vi "AFM_Driver_Manager.DestroyEvents.vi"(8 "error in (no error)":errorcluster, 11 "AFM_Driver_Manager in":refnum<class "AFM_Driver_Manager.lvclass">) -> (0 "error out":errorcluster, 3 "AFM_Driver_Manager out":refnum<class "AFM_Driver_Manager.lvclass">)   [LabVIEW 2019, in "AFM_Driver_Manager.lvclass"]
uses:
  AFM_Driver_Manager.lvclass
  AFM_Driver_Manager.lvclass/AFM_Driver_Manager.ctl
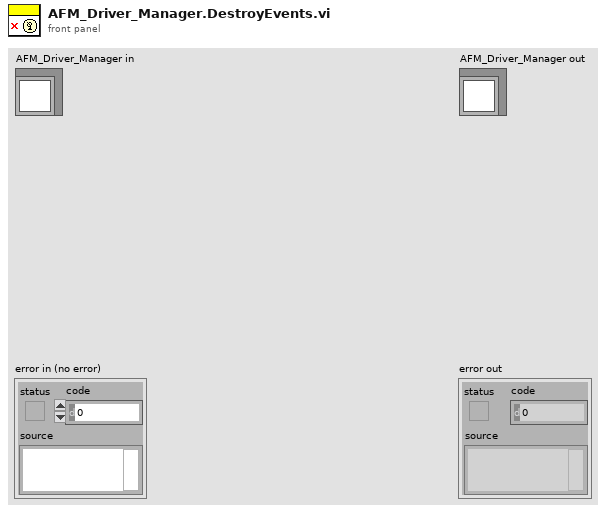
[diagram p1: front panel]
types:
  T1 = typedef "AFM_Driver_Manager.lvclass/AFM_Driver_Manager.PublicMethods.ctl" = cluster{"Stop Event":refnum<user-event>, "Lithography Data":refnum<user-event>, "Run Lithography":refnum<user-event>, "Background Image":refnum<user-event>, "Abort Notifier":refnum<user-event>}
  T2 = cluster{"VI Refnum":refnum<vi>, "Path":path, "Name":string, "Events":T1}[]
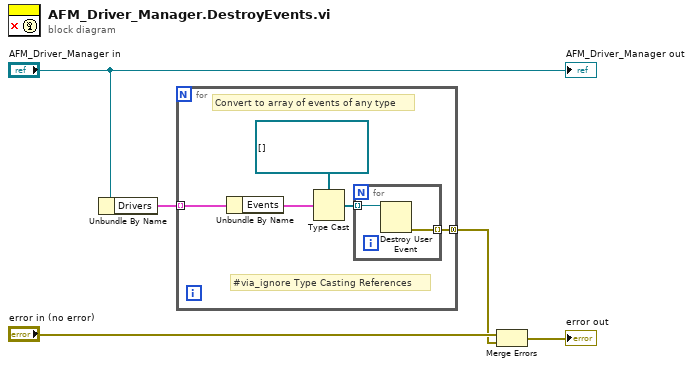
[diagram p0: block diagram]
diagram:
  n1 = Unbundle By Name("AFM_Driver_Manager in") -> ("Drivers"=w2:T2)
  n2 = for {
    tunnel: w2 -> [w10] mode=indexing
    tunnel: [w6] -> w1 mode=concatenating
    # "#via_ignore Type Casting References"
    # "Convert to array of events of any type"
    n3 = Unbundle By Name(w10) -> ("Events"=w8:T1)
    n4 = Type Cast(type=refnum<user-event>[] [], x=w8) -> (*(type *) &x=w7:refnum<user-event>[])
    n5 = for {
      tunnel: w7 -> [w12] mode=indexing
      tunnel: [w11] -> w6 mode=indexing
      n6 = Destroy User Event(user event=w12) -> (error out=w11:errorcluster)  [unwired: 1 in]
    }
  }
  n7 = Merge Errors("error in (no error)", w1) -> (→"error out":errorcluster)
  "AFM_Driver_Manager out" <- "AFM_Driver_Manager in"
